vi "Initiate (Immediate).vi"(8 "error in (no error)":errorcluster, 11 "VISA resource name":refnum<visa-resource-name>) -> (0 "error out":errorcluster, 3 "VISA resource name out":refnum<visa-resource-name>)   [LabVIEW 2014, in "Agilent U2000 Series.lvlib"]
doc: "Sets the U2000 Series power sensor in the wait for trigger state. When a trigger is received, the measurement is taken and the result placed in the U2000 Series power sensor memory. If Trigger Source is set to Immediate, the measurement begins as soon as this VI is executed."
uses:
  Agilent U2000 Series.lvlib
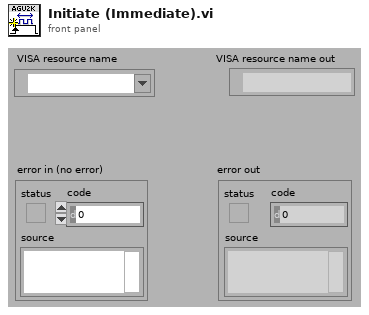
[diagram p1: front panel]
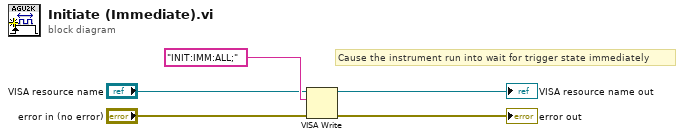
[diagram p0: block diagram]
diagram:
  # "Cause the instrument run into wait for trigger state immediately"
  n1 = VISA Write(VISA resource name="VISA resource name", write buffer="INIT:IMM:ALL;", error in (no error)="error in (no error)") -> (VISA resource name out=→"VISA resource name out":refnum<visa-resource-name>, error out=→"error out":errorcluster)  [unwired: 1 out]
